vi "SpectraPlot_QEPro.vi"(1 "array":dbl[](array[numeric])) -> (0 "output cluster":cluster{dbl[], dbl[]})   [LabVIEW 2016]
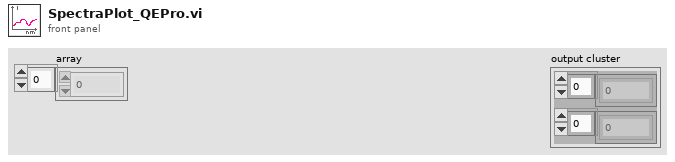
[diagram p1: front panel]
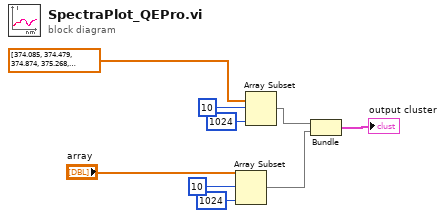
[diagram p0: block diagram]
diagram:
  n1 = Array Subset(array="array", index=10, length=1024) -> (w2:dbl[])
  n2 = Array Subset(array=dbl[] [374.085, 374.479, 374.874, 375.268, 375.663, 376.057, 376.452, 376.846, 377.24, 377.635, 378.029, 378.423, 378.817, 379.211, 379.605, 379.999, 380.393, 380.787, 381.181, 381.575, 381.969, 382.363, 382.756, 383.15, 383.544, 383.937, 384.331, 384.724, 385.118, 385.511, 385.905, 386.298, 386.691, 387.084, 387.478, 387.871, 388.264, 388.657, 389.05, 389.443, 389.836, 390.229, 390.622, 391.015, 391.408, 391.8, 392.193, 392.586, 392.978, 393.371, 393.764, 394.156, 394.549, 394.941, 395.333, 395.726, 396.118, 396.51, 396.902, 397.295, 397.687, 398.079, 398.471, 398.863, 399.255, 399.647, 400.039, 400.43, 400.822, 401.214, 401.606, 401.997, 402.389, 402.781, 403.172, 403.564, 403.955, 404.346, 404.738, 405.129, 405.52, 405.912, 406.303, 406.694, 407.085, 407.476, 407.867, 408.258, 408.649, 409.04, 409.431, 409.822, 410.213, 410.603, 410.994, 411.385, 411.775, 412.166, 412.556, 412.947, 413.337, 413.728, 414.118, 414.508, 414.899, 415.289, 415.679, 416.069, 416.459, 416.849, 417.239, 417.629, 418.019, 418.409, 418.799, 419.189, 419.579, 419.968, 420.358, 420.748, 421.137, 421.527, 421.916, 422.306, 422.695, 423.085, 423.474, 423.863, 424.252, 424.642, 425.031, 425.42, 425.809, 426.198, 426.587, 426.976, 427.365, 427.754, 428.143, 428.531, 428.92, 429.309, 429.697, 430.086, 430.475, 430.863, 431.252, 431.64, 432.029, 432.417, 432.805, 433.193, 433.582, 433.97, 434.358, 434.746, 435.134, 435.522, 435.91, 436.298, 436.686, 437.074, 437.462, 437.849, 438.237, 438.625, 439.012, 439.4, 439.788, 440.175, 440.563, 440.95, 441.337, 441.725, 442.112, 442.499, 442.886, 443.274, 443.661, 444.048, 444.435, 444.822, 445.209, 445.596, 445.983, 446.369, 446.756, 447.143, 447.53, 447.916, 448.303, 448.689, 449.076, 449.462, 449.849, 450.235, 450.622, 451.008, 451.394, 451.78, 452.166, 452.553, 452.939, 453.325, 453.711, 454.097, 454.483, 454.868, 455.254, 455.64, 456.026, 456.412, 456.797, 457.183, 457.568, 457.954, 458.339, 458.725, 459.11, 459.496, 459.881, 460.266, 460.651, 461.037, 461.422, 461.807, 462.192, 462.577, 462.962, 463.347, 463.732, 464.117, 464.501, 464.886, 465.271, 465.656, 466.04, 466.425, 466.809, 467.194, 467.578, 467.963, 468.347, 468.731, 469.116, 469.5, 469.884, 470.268, 470.652, 471.036, 471.42, 471.804, 472.188, 472.572, 472.956, 473.34, 473.724, 474.107, 474.491, 474.875, 475.258, 475.642, 476.025, 476.409, 476.792, 477.175, 477.559, 477.942, 478.325, 478.709, 479.092, 479.475, 479.858, 480.241, 480.624, 481.007, 481.39, 481.773, 482.155, 482.538, 482.921, 483.304, 483.686, 484.069, 484.451, 484.834, 485.216, 485.599, 485.981, 486.363, 486.746, 487.128, 487.51, 487.892, 488.274, 488.656, 489.038, 489.42, 489.802, 490.184, 490.566, 490.948, 491.33, 491.711, 492.093, 492.475, 492.856, 493.238, 493.619, 494.001, 494.382, 494.764, 495.145, 495.526, 495.907, 496.289, 496.67, 497.051, 497.432, 497.813, 498.194, 498.575, 498.956, 499.337, 499.717, 500.098, 500.479, 500.86, 501.24, 501.621, 502.001, 502.382, 502.762, 503.143, 503.523, 503.903, 504.284, 504.664, 505.044, 505.424, 505.804, 506.184, 506.564, 506.944, 507.324, 507.704, 508.084, 508.464, 508.844, 509.223, 509.603, 509.983, 510.362, 510.742, 511.121, 511.501, 511.88, 512.259, 512.639, 513.018, 513.397, 513.776, 514.156, 514.535, 514.914, 515.293, 515.672, 516.051, 516.43, 516.808, 517.187, 517.566, 517.945, 518.323, 518.702, 519.08, 519.459, 519.837, 520.216, 520.594, 520.973, 521.351, 521.729, 522.107, 522.486, 522.864, 523.242, 523.62, 523.998, 524.376, 524.754, 525.132, 525.509, 525.887, 526.265, 526.643, 527.02, 527.398, 527.775, 528.153, 528.53, 528.908, 529.285, 529.662, 530.04, 530.417, 530.794, 531.171, 531.548, 531.926, 532.303, 532.68, 533.056, 533.433, 533.81, 534.187, 534.564, 534.94, 535.317, 535.694, 536.07, 536.447, 536.823, 537.2, 537.576, 537.953, 538.329, 538.705, 539.081, 539.458, 539.834, 540.21, 540.586, 540.962, 541.338, 541.714, 542.09, 542.465, 542.841, 543.217, 543.593, 543.968, 544.344, 544.72, 545.095, 545.471, 545.846, 546.221, 546.597, 546.972, 547.347, 547.722, 548.098, 548.473, 548.848, 549.223, 549.598, 549.973, 550.348, 550.723, 551.097, 551.472, 551.847, 552.221, 552.596, 552.971, 553.345, 553.72, 554.094, 554.469, 554.843, 555.217, 555.592, 555.966, 556.34, 556.714, 557.088, 557.462, 557.836, 558.21, 558.584, 558.958, 559.332, 559.706, 560.079, 560.453, 560.827, 561.2, 561.574, 561.947, 562.321, 562.694, 563.068, 563.441, 563.814, 564.187, 564.561, 564.934, 565.307, 565.68, 566.053, 566.426, 566.799, 567.172, 567.545, 567.917, 568.29, 568.663, 569.036, 569.408, 569.781, 570.153, 570.526, 570.898, 571.271, 571.643, 572.015, 572.388, 572.76, 573.132, 573.504, 573.876, 574.248, 574.62, 574.992, 575.364, 575.736, 576.108, 576.479, 576.851, 577.223, 577.595, 577.966, 578.338, 578.709, 579.081, 579.452, 579.823, 580.195, 580.566, 580.937, 581.308, 581.679, 582.051, 582.422, 582.793, 583.164, 583.535, 583.905, 584.276, 584.647, 585.018, 585.388, 585.759, 586.13, 586.5, 586.871, 587.241, 587.612, 587.982, 588.352, 588.723, 589.093, 589.463, 589.833, 590.203, 590.573, 590.943, 591.313, 591.683, 592.053, 592.423, 592.793, 593.162, 593.532, 593.902, 594.271, 594.641, 595.01, 595.38, 595.749, 596.119, 596.488, 596.857, 597.227, 597.596, 597.965, 598.334, 598.703, 599.072, 599.441, 599.81, 600.179, 600.548, 600.917, 601.285, 601.654, 602.023, 602.391, 602.76, 603.128, 603.497, 603.865, 604.234, 604.602, 604.97, 605.338, 605.707, 606.075, 606.443, 606.811, 607.179, 607.547, 607.915, 608.283, 608.651, 609.018, 609.386, 609.754, 610.122, 610.489, 610.857, 611.224, 611.592, 611.959, 612.326, 612.694, 613.061, 613.428, 613.796, 614.163, 614.53, 614.897, 615.264, 615.631, 615.998, 616.365, 616.732, 617.098, 617.465, 617.832, 618.198, 618.565, 618.932, 619.298, 619.665, 620.031, 620.397, 620.764, 621.13, 621.496, 621.862, 622.229, 622.595, 622.961, 623.327, 623.693, 624.059, 624.425, 624.79, 625.156, 625.522, 625.888, 626.253, 626.619, 626.984, 627.35, 627.715, 628.081, 628.446, 628.812, 629.177, 629.542, 629.907, 630.272, 630.637, 631.003, 631.368, 631.733, 632.097, 632.462, 632.827, 633.192, 633.557, 633.921, 634.286, 634.651, 635.015, 635.38, 635.744, 636.109, 636.473, 636.837, 637.201, 637.566, 637.93, 638.294, 638.658, 639.022, 639.386, 639.75, 640.114, 640.478, 640.842, 641.205, 641.569, 641.933, 642.297, 642.66, 643.024, 643.387, 643.751, 644.114, 644.477, 644.841, 645.204, 645.567, 645.93, 646.293, 646.657, 647.02, 647.383, 647.745, 648.108, 648.471, 648.834, 649.197, 649.559, 649.922, 650.285, 650.647, 651.01, 651.372, 651.735, 652.097, 652.46, 652.822, 653.184, 653.546, 653.908, 654.271, 654.633, 654.995, 655.357, 655.719, 656.08, 656.442, 656.804, 657.166, 657.527, 657.889, 658.251, 658.612, 658.974, 659.335, 659.697, 660.058, 660.419, 660.781, 661.142, 661.503, 661.864, 662.225, 662.586, 662.947, 663.308, 663.669, 664.03, 664.391, 664.752, 665.112, 665.473, 665.834, 666.194, 666.555, 666.915, 667.276, 667.636, 667.996, 668.357, 668.717, 669.077, 669.437, 669.798, 670.158, 670.518, 670.878, 671.238, 671.597, 671.957, 672.317, 672.677, 673.037, 673.396, 673.756, 674.115, 674.475, 674.834, 675.194, 675.553, 675.912, 676.272, 676.631, 676.99, 677.349, 677.708, 678.067, 678.427, 678.785, 679.144, 679.503, 679.862, 680.221, 680.58, 680.938, 681.297, 681.655, 682.014, 682.372, 682.731, 683.089, 683.448, 683.806, 684.164, 684.522, 684.881, 685.239, 685.597, 685.955, 686.313, 686.671, 687.029, 687.386, 687.744, 688.102, 688.46, 688.817, 689.175, 689.532, 689.89, 690.247, 690.605, 690.962, 691.32, 691.677, 692.034, 692.391, 692.748, 693.105, 693.463, 693.82, 694.176, 694.533, 694.89, 695.247, 695.604, 695.961, 696.317, 696.674, 697.03, 697.387, 697.743, 698.1, 698.456, 698.813, 699.169, 699.525, 699.881, 700.237, 700.594, 700.95, 701.306, 701.662, 702.017, 702.373, 702.729, 703.085, 703.441, 703.796, 704.152, 704.508, 704.863, 705.219, 705.574, 705.929, 706.285, 706.64, 706.995, 707.351, 707.706, 708.061, 708.416, 708.771, 709.126, 709.481, 709.836, 710.191, 710.545, 710.9, 711.255, 711.609, 711.964, 712.319, 712.673, 713.028, 713.382, 713.736, 714.091, 714.445, 714.799, 715.153, 715.507, 715.862, 716.216, 716.57, 716.923, 717.277, 717.631, 717.985, 718.339, 718.692, 719.046, 719.4, 719.753, 720.107, 720.46, 720.814, 721.167, 721.52, 721.874, 722.227, 722.58, 722.933, 723.286, 723.639, 723.992, 724.345, 724.698, 725.051, 725.404, 725.757, 726.109, 726.462, 726.815, 727.167, 727.52, 727.872, 728.225, 728.577, 728.929, 729.282, 729.634, 729.986, 730.338, 730.69, 731.042, 731.394, 731.746, 732.098, 732.45, 732.802, 733.153, 733.505, 733.857, 734.208, 734.56, 734.912, 735.263, 735.614, 735.966, 736.317, 736.668, 737.02, 737.371, 737.722, 738.073, 738.424, 738.775, 739.126, 739.477, 739.828, 740.179, 740.529, 740.88, 741.231, 741.581, 741.932, 742.283, 742.633, 742.983, 743.334, 743.684, 744.034, 744.385, 744.735, 745.085, 745.435, 745.785, 746.135, 746.485, 746.835, 747.185, 747.535, 747.884, 748.234, 748.584, 748.933, 749.283, 749.632, 749.982, 750.331, 750.681, 751.03, 751.379, 751.729, 752.078, 752.427, 752.776, 753.125, 753.474, 753.823, 754.172, 754.521, 754.87, 755.218, 755.567, 755.916, 756.264, 756.613, 756.961, 757.31, 757.658, 758.007, 758.355, 758.703, 759.051, 759.4, 759.748, 760.096, 760.444, 760.792, 761.14, 761.488, 761.836] ("all rows"), index=10, length=1024) -> (w3:dbl[])
  n3 = Bundle(w3, w2) -> (→"output cluster":cluster{dbl[], dbl[]})  [unwired: 1 in]
